vi "Global_data.vi"() -> ()   [LabVIEW 2018]
panel:
  in  "global 2d graph":dbl[][](array[numeric])
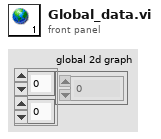
[diagram p1: front panel]
diagram:
